vi "registration-test.vi"(8 "error in (no error)":errorcluster) -> (0 "error out":errorcluster)   [LabVIEW 2021]
uses:
  <vilib>/addons/_JKI Toolkits/Caraya/classes/Test/Test.lvclass
  src/SMO/SMO.lvclass
  src/Registry/Registry-SMO.lvclass
  <vilib>/addons/_JKI Toolkits/Caraya/classes/Assert/Assert.lvclass
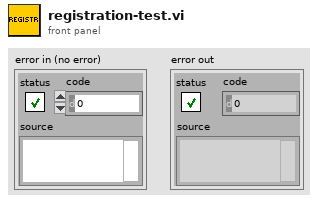
[diagram p1: front panel]
types:
  T1 = typedef "smo.lvlib/Registry-SMO.lvclass/PublicRegistryEvents--Cluster.ctl" = cluster{"Register Event":refnum<user-event>, "Unregister Event":refnum<user-event>}
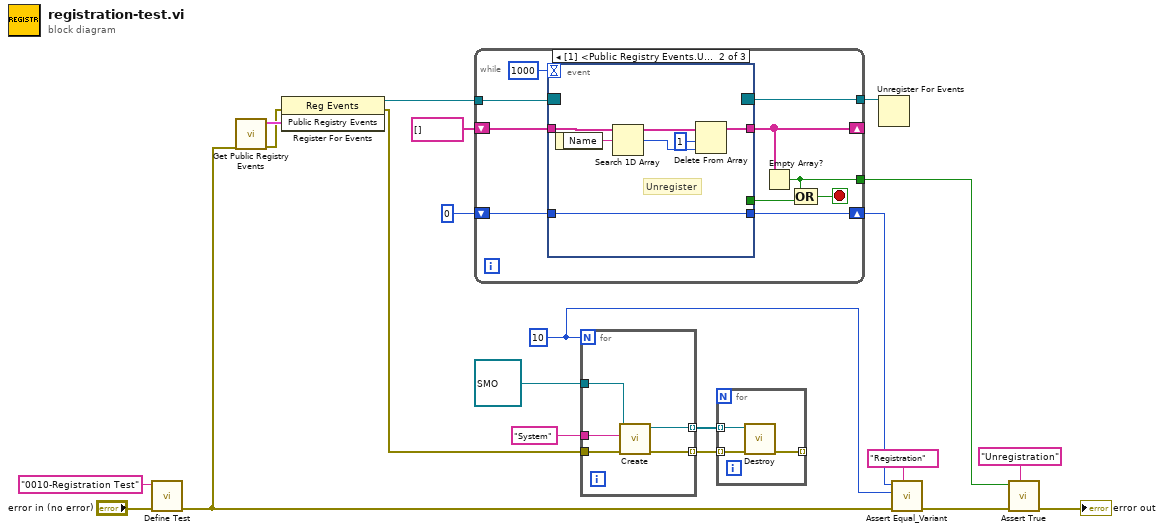
[diagram p0: block diagram]
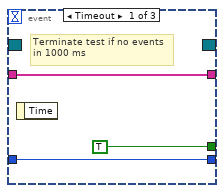
[diagram p2: hidden frame]
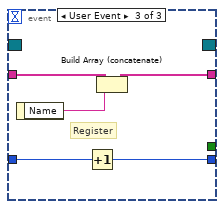
[diagram p3: hidden frame]
diagram:
  w6 = 10
  n1 = call <vilib>:"Define Test.vi"("error in (no error)"="error in (no error)", "Label (VI Title)"="0010-Registration Test") -> ("error out"=w9:errorcluster)  [unwired: 9 in]
  n2 = call "Get Public Registry Events.vi"("error in (no error)"=w9) -> ("error out"=w10:errorcluster, "Public Registry Events"=w18:T1)  [unwired: 9 in]
  n3 = register-events(error in=w10, w18) -> (reference out=w17:refnum<event-registration>, error out=w11:errorcluster)  [unwired: 1 in]
  n4 = while {
    tunnel: w17 -> [w31]
    shift-right: [w29] -> _
    shift-left: string[] [] -> [w30]
    tunnel: [w28] -> w15
    shift-right: [w27] -> w7
    shift-left: 0 -> [w26]
    tunnel: [w22] -> w3
    stop <- w23 stop-if-true
    n5 = event shown="[1] <Public Registry Events.Unregister Event>: User Event" {
      selector: w31 -> [_ _ _]
      dyn-events: [_ _ _] -> w28
      timeout: 1000 -> [_ _ _]
      tunnel: w30 -> [w34 w39 w45]
      tunnel: [w34 w38 w43] -> w29
      tunnel: [w33 w35 w42] -> w27
      tunnel: w26 -> [w33 w35 w41]
      tunnel: [TRUE _ _] -> w24
      event Timeout {
        # "Terminate test if no events\nin 1000 ms"
        n6 = event-data() -> ()  [unwired: 1 in, 1 out]
      }
      event User Event {
        # "Unregister"
        n7 = event-data() -> ("Name"=w40:string)  [unwired: 1 in]
        n8 = Search 1D Array(1D array=w39, element=w40) -> (index of element=w37:i32)  [unwired: 1 in]
        n9 = Delete From Array(array=w39, length=1, index=w37) -> (array with subset deleted=w38:string[])  [unwired: 1 out]
      }
      event User Event {
        # "Register"
        n10 = event-data() -> ("Name"=w44:string)  [unwired: 1 in]
        n11 = Increment(x=w41) -> (x+1=w42:i32)
        n12 = Build Array (concatenate)(w45, w44) -> (w43:string[])
      }
    }
    n13 = Empty Array?(array=w29) -> (empty?=w22:bool)
    n14 = Compound Arithmetic op=OR(w22, w24) -> (w23:bool)
  }
  n15 = for {
    N: w6 -> [_]
    tunnel: "System" ("Subsystem Name (optional)") -> [w50]
    tunnel: [w49] -> w13 mode=indexing
    tunnel: [w48] -> w12 mode=indexing
    tunnel: w11 -> [w47]
    tunnel: refnum<class "SMO.lvclass"> refnum ("Dependency Type") -> [w46]
    n16 = call "Create.vi"("error in (no error)"=w47, "Subsystem Name (optional)"=w50, "SMO"=w46) -> ("error out"=w48:errorcluster, "SMO out"=w49:refnum<class "SMO.lvclass">)  [unwired: 6 in, 1 out]
  }
  n17 = for {
    tunnel: w13 -> [w53] mode=indexing
    tunnel: [w52] -> _ mode=indexing
    tunnel: w12 -> [w51] mode=indexing
    n18 = call "Destroy.vi"("error in (no error)"=w51, "SMO"=w53) -> ("error out"=w52:errorcluster)  [unwired: 9 in]
  }
  n19 = Unregister For Events(event registration refnum=w15) -> ()  [unwired: 1 in, 1 out]
  n20 = call <vilib>:"Assert Equal_Variant.vi"("Label"="Registration" ("Label (VI Title)"), "error in (no error)"=w9, "Y"=w6, "X"=w7) -> ("error out"=w5:errorcluster)  [unwired: 7 in]
  n21 = call <vilib>:"Assert True.vi"("Label"="Unregistration" ("Label (VI Title)"), "error in (no error)"=w5, "True?"=w3) -> ("error out"=→"error out":errorcluster)  [unwired: 8 in]
